vi "SerialNumber.vi"() -> ()   [LabVIEW 2012]
panel:
  in  "SerialNumber":string
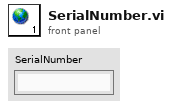
[diagram p1: front panel]
diagram:
